vi "GetType.vi"(8 "error in (no error)":errorcluster, 11 "Configure RangeMax Msg":refnum<class "Configure RangeMax Msg.lvclass">) -> (0 "error out":errorcluster, 2 "Data Sample":variant, 3 "Configure RangeMax Msg":refnum<class "Configure RangeMax Msg.lvclass">)   [LabVIEW 2015, in "CS++Motor.lvlib" / "Configure RangeMax Msg.lvclass"]
uses:
  Configure RangeMax Msg.lvclass
  Configure RangeMax Msg.lvclass/Configure RangeMax Msg.ctl
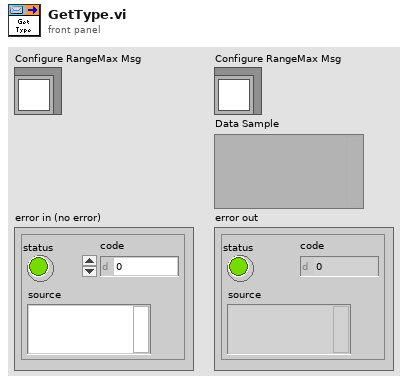
[diagram p1: front panel]
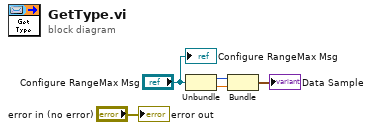
[diagram p0: block diagram]
diagram:
  n1 = Unbundle("Configure RangeMax Msg") -> (w2:u8, w1:dbl)
  n2 = Bundle("AxisNumber"=w2, "RangeMax"=w1) -> (→"Data Sample":cluster{"AxisNumber":u8, "RangeMax":dbl})  [unwired: 1 in]
  "error out" <- "error in (no error)"
  "Configure RangeMax Msg" <- "Configure RangeMax Msg"
